vi "Level Meter Control Panel (No Objects).vi"(8 "error in (no error)":errorcluster) -> (0 "error out":errorcluster)   [LabVIEW 2017]
uses:
  Cryogen Levels.ctl
  Oxford/BUSGEN.LLB/OxfordAddress.ctl
  Utility Classes/Readable/Readable.lvclass
  Level Meter.lvclass
panel:
  in  "danger":string="Sound\\Voice\\danger.wav"
  out "*ilm200 (No Ob)":T3={"helium"={"fastHe?"=FALSE, "slowHe?"=FALSE, "fillHe?"=FALSE, "lowHe?"=FALSE}, "nitrogen"={"fillN?"=FALSE, "lowN?"=FALSE}, "Shutdown"=FALSE, "Cryogen Levels"=[], "IO Info"={"Address"={"Com Port"=1, "ISOBUS Address"=5, "GPIB Address"=24, "Communication"=enum."ISOBUS"}, "ILM Name"="", "Display Channel"=[]}} {"Cryogen Levels" min=-1.0 max=100.0 scale=0.0..100.0}
  in  "Cluster In":T3={"helium"={"fastHe?"=FALSE, "slowHe?"=FALSE, "fillHe?"=FALSE, "lowHe?"=FALSE}, "nitrogen"={"fillN?"=FALSE, "lowN?"=FALSE}, "Shutdown"=FALSE, "Cryogen Levels"=[], "IO Info"={"Address"={"Com Port"=1, "ISOBUS Address"=5, "GPIB Address"=24, "Communication"=enum."ISOBUS"}, "ILM Name"="", "Display Channel"=[]}} {"Cryogen Levels" min=-1.0 max=100.0 scale=0.0..100.0}
  out "Log Counter":dbl
  out "Alarm":bool
  in  "Display last":dbl[unit]=600.0
  out "TX graph":T4(graph)
  in  "Update interval":dbl[unit]=0.1
  in  "Internal UI Refresh":bool
  out "done?":bool
  out "Heliters":dbl caption="LHe Liters" format="%.3f"
  in  "Fast? He":bool
  in  "warningcontN":T5={"alarmliqN"=90.0, "warn?N"=FALSE, "lessthan?N"=FALSE}
  in  "warningcontHe":T6={"alarmliqHe"=85.0, "warn?He"=FALSE, "lessthan?He"=FALSE}
  out "Cryogen Levels":T1 min=-1.0 max=100.0 scale=0.0..100.0
  out "helium":T7 caption="Helium"
  out "nitrogen":cluster{"fillN?":bool, "lowN?":bool} caption="Nitrogen"
  out "shutdown":bool caption="Shut Down"
  out "active":bool
  out "working":bool caption="Working"
  out "ready?":bool
  in  "Refresh":bool
  in  "endprgm":bool
  # "Level Meter Control Panel"
  # "Helium"
  # "Cryogen Levels"
  # "Warning"
  # "Nitrogen"
  # "L"
  # "He Sample Rate"
  # "Slow"
  # "Fast"
  # "Off"
  # "On"
  # "Greater"
  # "Less"
  # "Off"
  # "On"
  # "Greater"
  # "Less"
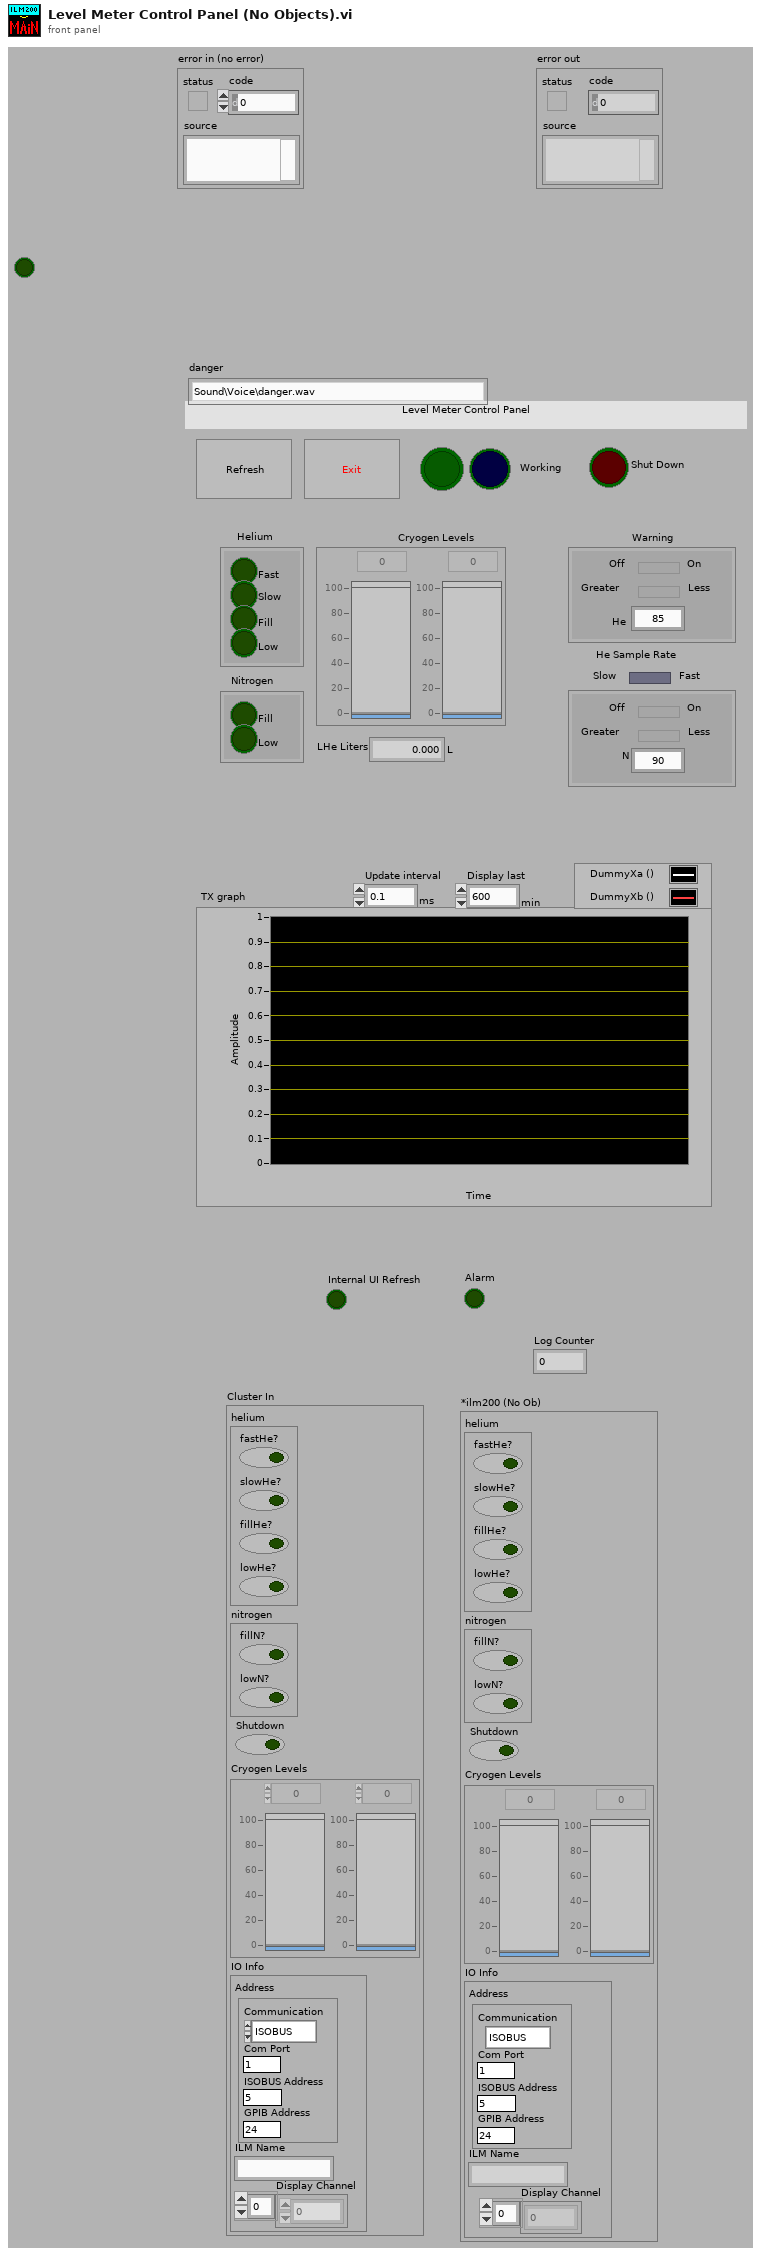
[diagram p1: front panel]
types:
  T1 = typedef "Level Meter.lvclass/Cryogen Levels.ctl" = dbl[]
  T2 = typedef "OxfordAddress.ctl" = cluster{"Com Port":i32, "ISOBUS Address":i32, "GPIB Address":i16, "Communication":enum16{"RS232", "ISOBUS", "GPIB", "Gateway"}}
  T3 = cluster{"helium":cluster{"fastHe?":bool, "slowHe?":bool, "fillHe?":bool, "lowHe?":bool}, "nitrogen":cluster{"fillN?":bool, "lowN?":bool}, "Shutdown":bool, "Cryogen Levels":T1, "IO Info":cluster{"Address":T2, "ILM Name":string, "Display Channel":i32[]}}
  T4 = cluster{"Data Points":cluster{"t":timestamp, "x":dbl}[]}[]
  T5 = cluster{"alarmliqN":dbl, "warn?N":bool, "lessthan?N":bool}
  T6 = cluster{"alarmliqHe":dbl, "warn?He":bool, "lessthan?He":bool}
  T7 = cluster{"fastHe?":bool, "slowHe?":bool, "fillHe?":bool, "lowHe?":bool}
  T8 = typedef "Readable.lvclass/TX Graph.ctl" = cluster{"Data Points":cluster{"t":timestamp, "x":dbl}[]}[]
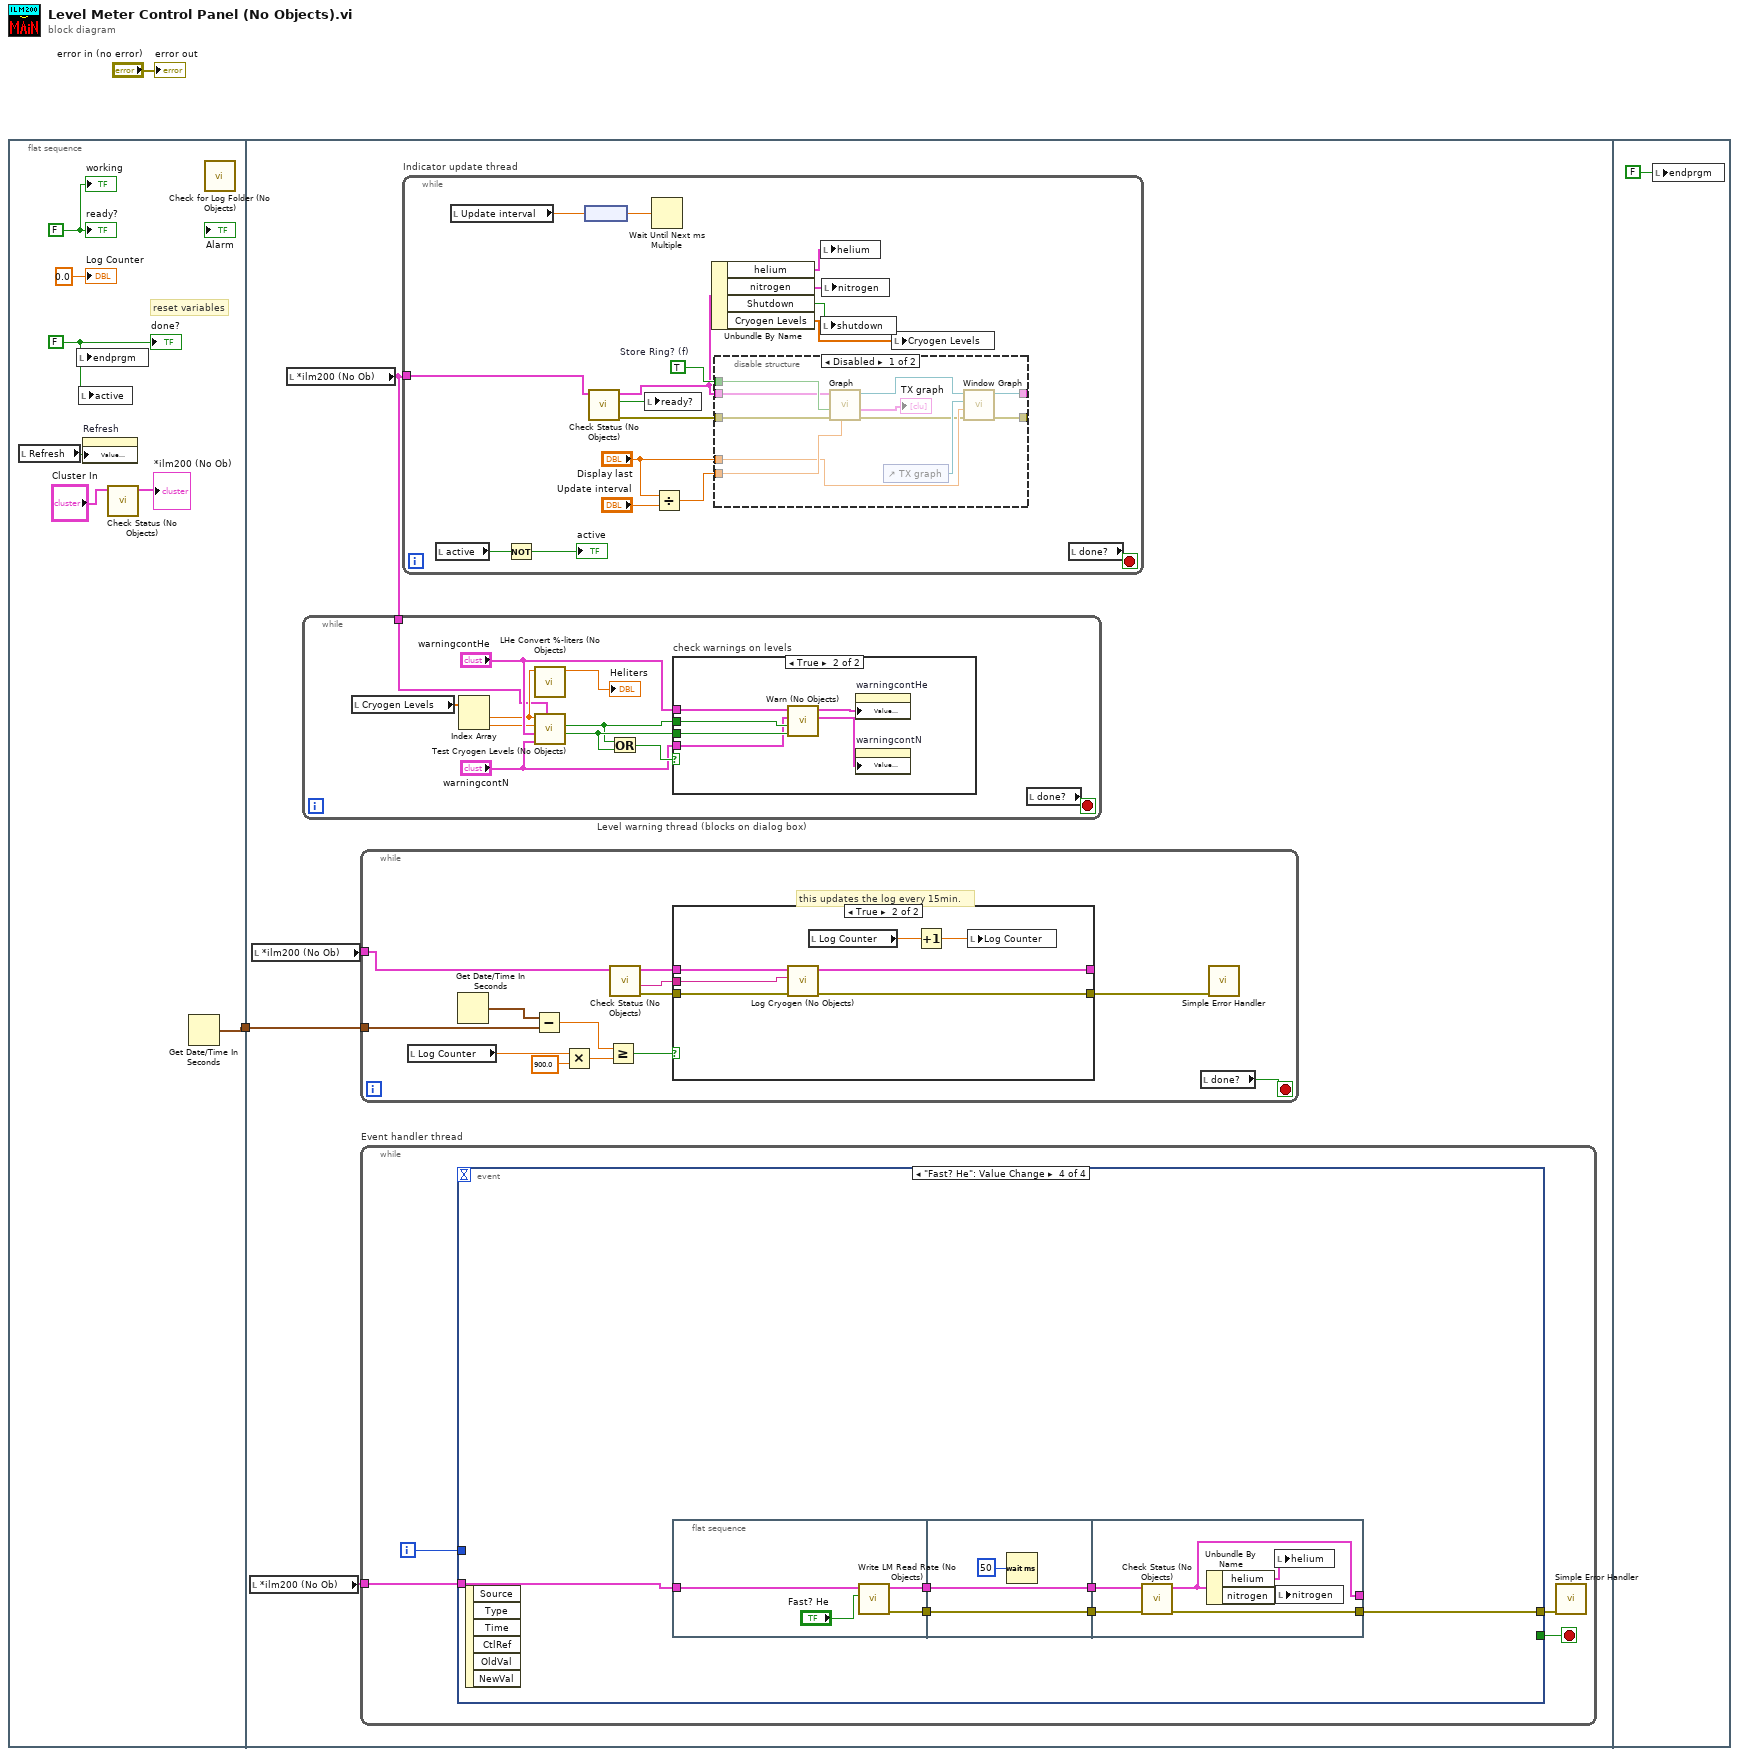
[diagram p0: block diagram]
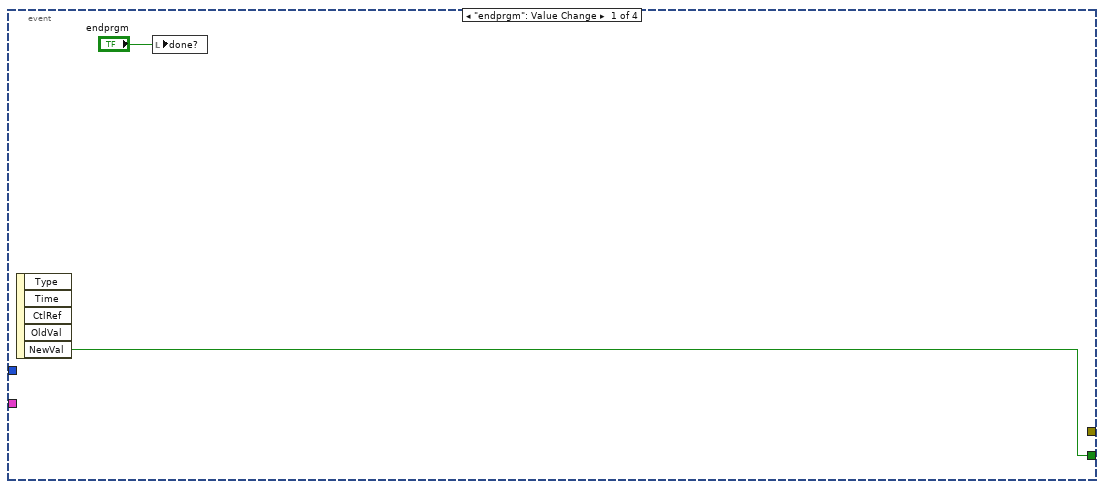
[diagram p5: hidden frame]
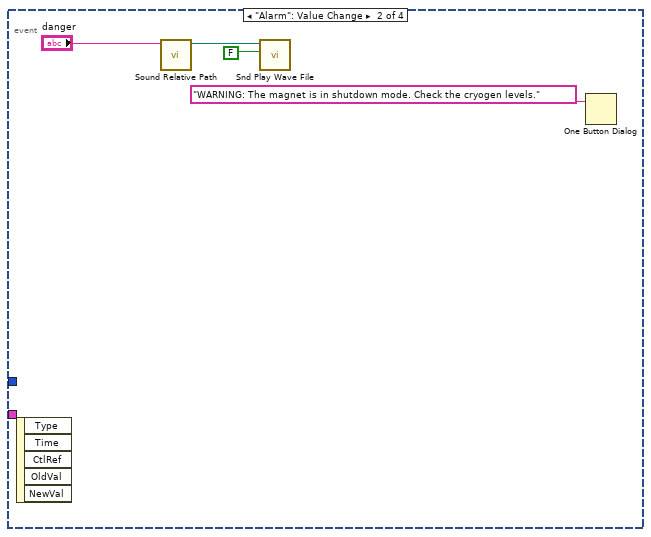
[diagram p6: hidden frame]
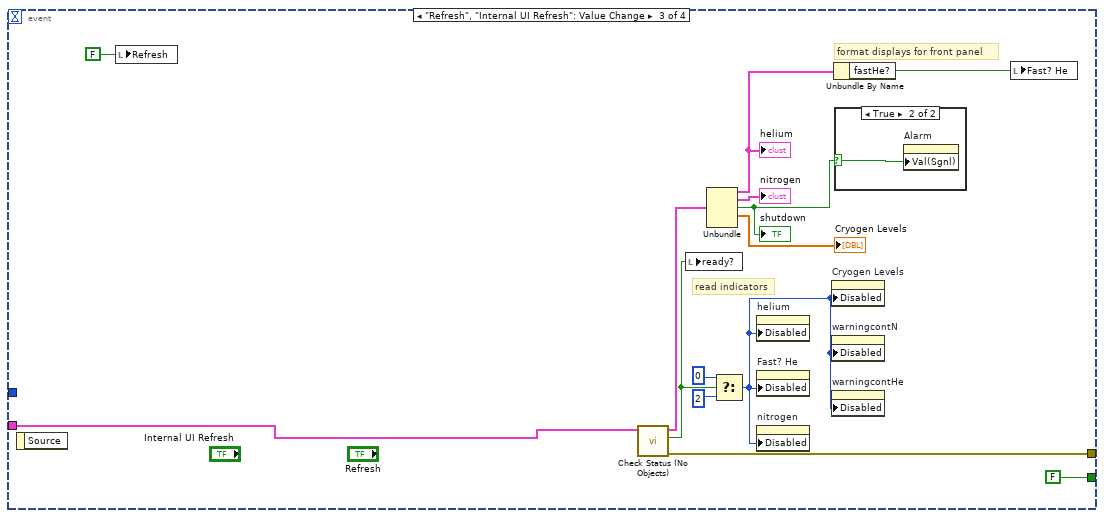
[diagram p7: hidden frame]
diagram:
  n1 = flat-sequence {
    tunnel: [w6] -> w1
    tunnel: w1 -> [w13]
    frame #0 {
      w9 = FALSE
      w7 = FALSE
      # "reset variables"
      n2 = local read "Refresh"() -> (w8:bool)
      n3 = local write "endprgm"(w7) -> ()
      n4 = local write "active"(w7) -> ()
      n5 = property on="Refresh" class="Bool (strict)"("Value (Signaling)"=w8) -> ()  [unwired: 2 in, 2 out]
      n6 = call "Check Status (No Objects).vi"("Cluster In"="Cluster In") -> ("Cluster Out"=→"*ilm200 (No Ob)":T3)  [unwired: 7 in, 3 out]
      n7 = Get Date/Time In Seconds() -> (seconds since 1Jan1904=w6:timestamp)
      n8 = call "Check for Log Folder (No Objects).vi"() -> ()  [unwired: 1 in]
      "ready?" <- w9
      "working" <- w9
      "done?" <- w7
      "Log Counter" <- 0.0 ("Log Counter")
    }
    frame #1 {
      n9 = local read "*ilm200 (No Ob)"() -> (w10:T3)
      n10 = local read "*ilm200 (No Ob)"() -> (w12:T3)
      n11 = local read "*ilm200 (No Ob)"() -> (w11:T3)
      n12 = while "Level warning thread (blocks on dialog box)" {
        tunnel: w11 -> [w36]
        stop <- w37 stop-if-true
        n13 = local read "Cryogen Levels"() -> (w38:T1)
        n14 = Index Array(array=w38) -> (element #1=w40:dbl, element #2=w39:dbl)  [unwired: 2 in]
        n15 = call "LHe Convert %-liters (No Objects).vi"("%"=w40) -> ("Lout"=→"Heliters":dbl)  [unwired: 9 in, 1 out]
        n16 = call "Test Cryogen Levels (No Objects).vi"("Cluster In"=w36, "warningcontN"="warningcontN", "warningcontHe"="warningcontHe", "LNlevel"=w39, "LHelevel"=w40) -> ("warnN"=w45:bool, "warnHe"=w44:bool)  [unwired: 4 in, 1 out]
        n17 = Or(x=w44, y=w45) -> (x .or. y?=w43:bool)
        n18 = case "check warnings on levels" shown="True" w43 {
          tunnel: w44 -> [_ w52]
          tunnel: w45 -> [_ w51]
          tunnel: "warningcontHe" -> [_ w50]
          tunnel: "warningcontN" -> [_ w49]
          frame False {
          }
          frame True {
            n19 = call "Warn (No Objects).vi"("NwarnIN"=w51, "HwarnIN"=w52, "warncontN"=w49, "warncontHe"=w50) -> ("warnNOUT"=w48:T5, "warnHeOUT"=w47:T6)  [unwired: 6 in]
            n20 = property on="warningcontHe" class="Clust (strict)"("Value (Signaling)"=w47) -> ()  [unwired: 2 in, 2 out]
            n21 = property on="warningcontN" class="Clust (strict)"("Value (Signaling)"=w48) -> ()  [unwired: 2 in, 2 out]
          }
        }
        n22 = local read "done?"() -> (w37:bool)
      }
      n23 = while {
        tunnel: w12 -> [w14]
        tunnel: w13 -> [w20]
        stop <- w26 stop-if-true
        # "this updates the log every 15min."
        n24 = local read "Log Counter"() -> (w18:dbl)
        n25 = Get Date/Time In Seconds() -> (seconds since 1Jan1904=w21:timestamp)
        n26 = Subtract(x=w21, y=w20) -> (x-y=w17:dbl)
        n27 = Multiply(x=w18, y=900.0 ("millisecond multiple")) -> (x*y=w16:dbl)
        n28 = Greater Or Equal?(x=w17, y=w16) -> (x >= y?=w22:bool)
        n29 = call "Check Status (No Objects).vi"("Cluster In"=w14) -> ("error out"=w25:errorcluster, "Status"=w24:string, "Cluster Out"=w23:T3)  [unwired: 7 in, 1 out]
        n30 = case shown="True" w22 {
          tunnel: w25 -> [w27 w35]
          tunnel: w24 -> [_ w34]
          tunnel: w23 -> [w28 w29]
          tunnel: [w27 w33] -> w15
          tunnel: [w28 w32] -> _
          frame False {
          }
          frame True {
            n31 = call "Log Cryogen (No Objects).vi"("error in (no error)"=w35, "Status string"=w34, "Cluster In"=w29) -> ("error out"=w33:errorcluster, "Cluster Out"=w32:T3)  [unwired: 7 in]
            n32 = local read "Log Counter"() -> (w31:dbl)
            n33 = Increment(x=w31) -> (x+1=w30:dbl)
            n34 = local write "Log Counter"(w30) -> ()
          }
        }
        n35 = local read "done?"() -> (w26:bool)
        n36 = call <vilib>:"Simple Error Handler.vi"("error in (no error)"=w15) -> ()  [unwired: 4 in, 5 out]
      }
      n37 = while "Event handler thread" {
        tunnel: w10 -> [w84]
        i -> [w85]
        stop <- w86 stop-if-true
        n38 = event shown="[3] \"Fast? He\": Value Change" {
          selector: _ -> [_ _ _ _]
          dyn-events: _ -> [_ _ _ _]
          timeout: _ -> [_ _ _ _]
          tunnel: [w88 _ FALSE _] -> w86
          tunnel: w85 -> [_ _ _ _]
          tunnel: w84 -> [_ _ w93 w108]
          tunnel: [_ _ w94 w109] -> w83
          event "endprgm": Value Change {
            n39 = event-data() -> ("NewVal"=w88:bool)  [unwired: 5 out]
            n40 = local write "done?"("endprgm") -> ()
          }
          event "Alarm": Value Change {
            n41 = event-data() -> ()  [unwired: 6 out]
            n42 = call "Sound Relative Path.vi"("Sound"="danger") -> ("Relative Path"=w91:path)  [unwired: 10 in]
            n43 = call <vilib>:"Snd Play Wave File.vi"("wait until finish (T)"=FALSE, "wave file path"=w91) -> ()  [unwired: 1 in, 9 out]
            n44 = One Button Dialog(message="WARNING: The magnet is in shutdown mode. Check the cryogen levels.") -> ()  [unwired: 1 in, 1 out]
          }
          event "Refresh", "Internal UI Refresh": Value Change {
            # "format displays for front panel"
            # "read indicators"
            n45 = event-data() -> ()  [unwired: 2 out]
            n46 = local write "Refresh"(FALSE) -> ()
            n47 = call "Check Status (No Objects).vi"("Cluster In"=w93) -> ("error out"=w94:errorcluster, "On?"=w101:bool, "Cluster Out"=w96:T3)  [unwired: 7 in, 1 out]
            n48 = local write "ready?"(w101) -> ()
            n49 = Unbundle(w96) -> ("helium"=w98:T7, "nitrogen"=→"nitrogen":cluster{"fillN?":bool, "lowN?":bool}, "Shutdown"=w95:bool, "Cryogen Levels"=→"Cryogen Levels":T1)  [unwired: 1 out]
            "helium" <- w98
            "shutdown" <- w95
            n50 = Select(t=0, s=w101, f=2) -> (s? t:f=w102:i32)
            n51 = property on="helium" class="Clust (strict)"("Disabled"=w102) -> ()  [unwired: 2 in, 2 out]
            n52 = property on="Fast? He" class="Bool (strict)"("Disabled"=w102) -> ()  [unwired: 2 in, 2 out]
            n53 = property on="nitrogen" class="Clust (strict)"("Disabled"=w102) -> ()  [unwired: 2 in, 2 out]
            n54 = property on="Cryogen Levels" class="Arr (strict)"("Disabled"=w102) -> ()  [unwired: 2 in, 2 out]
            n55 = property on="warningcontN" class="Clust (strict)"("Disabled"=w102) -> ()  [unwired: 2 in, 2 out]
            n56 = property on="warningcontHe" class="Clust (strict)"("Disabled"=w102) -> ()  [unwired: 2 in, 2 out]
            n57 = Unbundle By Name(w98) -> ("fastHe?"=w97:bool)
            n58 = case shown="True" w95 {
              selector: w95 -> [_ w107]
              frame False {
              }
              frame True {
                n59 = property on="Alarm" class="Bool (strict)"("Val(Sgnl)"=w107) -> ()  [unwired: 2 in, 2 out]
              }
            }
            n60 = local write "Fast? He"(w97) -> ()
          }
          event "Fast? He": Value Change {
            n61 = event-data() -> ()  [unwired: 7 out]
            n62 = flat-sequence {
              tunnel: [w116] -> w113
              tunnel: [w115] -> w110
              tunnel: w108 -> [w114]
              tunnel: w113 -> [w119]
              tunnel: [w119] -> w112
              tunnel: [w118] -> w111
              tunnel: w110 -> [w118]
              tunnel: [w124] -> _
              tunnel: w112 -> [w121]
              tunnel: w111 -> [w123]
              tunnel: [w122] -> w109
              frame #0 {
                n63 = call "Write LM Read Rate (No Objects).vi"("Fast?"="Fast? He", "Cluster In"=w114) -> ("error out"=w115:errorcluster, "Cluster Out"=w116:T3)  [unwired: 8 in]
              }
              frame #1 {
                n64 = Wait (ms)(milliseconds to wait=50) -> ()  [unwired: 1 out]
              }
              frame #2 {
                n65 = call "Check Status (No Objects).vi"("error in (no error)"=w123, "Cluster In"=w121) -> ("error out"=w122:errorcluster, "Cluster Out"=w124:T3)  [unwired: 6 in, 2 out]
                n66 = Unbundle By Name(w124) -> ("helium"=w126:T7, "nitrogen"=w125:cluster{"fillN?":bool, "lowN?":bool})
                n67 = local write "helium"(w126) -> ()
                n68 = local write "nitrogen"(w125) -> ()
              }
            }
          }
        }
        n69 = call <vilib>:"Simple Error Handler.vi"("error in (no error)"=w83) -> ()  [unwired: 4 in, 5 out]
      }
      n70 = while "Indicator update thread" {
        tunnel: w11 -> [w53]
        stop <- w56 stop-if-true
        w69 = TRUE  # Store Ring? (f)
        n71 = local read "active"() -> (w62:bool)
        n72 = local read "Update interval"() -> (w64:dbl[unit])
        n73 = Not(x=w62) -> (.not. x?=→"active":bool)
        n74 = node(w64) -> (w68:dbl)
        n75 = call "Check Status (No Objects).vi"("Cluster In"=w53) -> ("error out"=w54:errorcluster, "On?"=w57:bool, "Cluster Out"=w55:T3)  [unwired: 7 in, 1 out]
        n76 = local write "ready?"(w57) -> ()
        n77 = Wait Until Next ms Multiple(millisecond multiple=w68) -> ()  [unwired: 1 out]
        n78 = Divide(x="Display last", y="Update interval") -> (x/y=w66:dbl)
        n79 = Unbundle By Name(w55) -> ("helium"=w58:T7, "nitrogen"=w60:cluster{"fillN?":bool, "lowN?":bool}, "Shutdown"=w59:bool, "Cryogen Levels"=w61:T1)
        n80 = disable-structure shown="Disabled" {
          disable-tunnel: w69 -> [w80 _]
          disable-tunnel: w66 -> [w78 _]
          disable-tunnel: "Display last" -> [w77 _]
          disable-tunnel: w55 -> [w73 w82]
          disable-tunnel: w54 -> [w72 w81]
          disable-tunnel: [w71 w82] -> _
          disable-tunnel: [w70 w81] -> _
          frame Disabled {
            n81 = call-dynamic "Graph.vi"("Ring size (points) (1024)"=w78, "error in (no error)"=w72, "Store Ring? (f)"=w80, "Readable in"=w73) -> ("error out"=w74:errorcluster, "Ring Buffers"=→"TX graph":T8, "Readable out"=w75:refnum<class "Readable.lvclass">)  [unwired: 3 in, 2 out]
            n82 = control-ref of="TX graph"() -> (w76:refnum<vi>)
            n83 = call-dynamic "Window Graph.vi"("error in (no error)"=w74, "Window"=w77, "Graph ref"=w76, "Readable in"=w75) -> ("error out"=w70:errorcluster, "Readable out"=w71:refnum<class "Readable.lvclass">)  [unwired: 6 in]
          }
          frame Enabled {
          }
        }
        n84 = local write "helium"(w58) -> ()
        n85 = local write "shutdown"(w59) -> ()
        n86 = local write "nitrogen"(w60) -> ()
        n87 = local write "Cryogen Levels"(w61) -> ()
        n88 = local read "done?"() -> (w56:bool)
      }
    }
    frame #2 {
      n89 = local write "endprgm"(FALSE) -> ()
    }
  }
  "error out" <- "error in (no error)"
